vi "cm2nm_write_session_file.vi"(1 "Session Information":T1) -> (0 "NaN/Path/Refnum?":bool)   [LabVIEW 2011]
doc: "Write the session information to xml file, path contained in the field internal field \"CollectionFile\"."
uses:
  cm2nm_sample_set.ctl
  cm2nm_coordinate_information_v2.ctl
  Instrument_type_enum_v2.ctl
  <vilib>/Utility/xml.llb/Write to XML File(string).vi
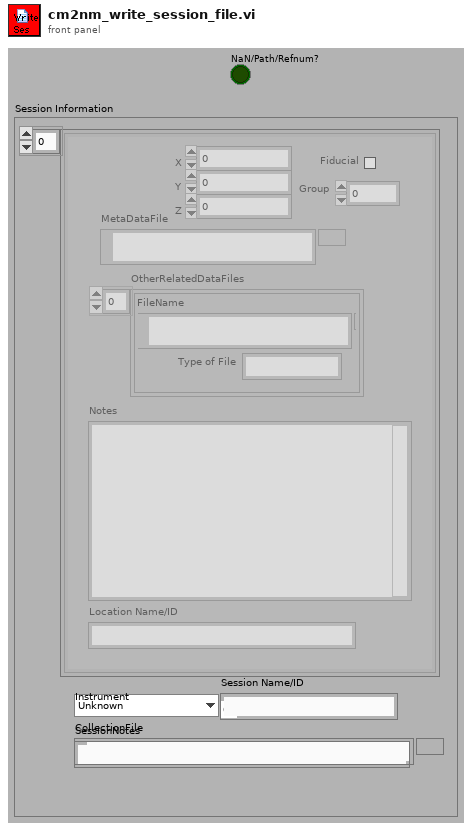
[diagram p1: front panel]
types:
  T1 = typedef "cm2nm_sample_set.ctl" = cluster{"CollectionOfPoints":T2[], "Instrument":T3, "CollectionFile":path, "Session Name/ID":string, "SessionNotes":string}
  T2 = typedef "cm2nm_coordinate_information_v2.ctl" = cluster{"MetaDataFile":path, "X":dbl, "Y":dbl, "Z":dbl, "Group":i32, "Rotation":dbl[unit], "Fiducial":bool, "Magnification":dbl, "Working_Distance":dbl, "Notes":string, "Location Name/ID":string, "OtherRelatedDataFiles":cluster{"Type of File":string, "FileName":path}[], "Available":bool}
  T3 = typedef "Instrument_type_enum_v2.ctl" = enum16{"Unknown", "Philips FEI SEM IRC", "JEOL 7000F EML_MFC", "MXRD MFC", "JEOL_EPMA"}
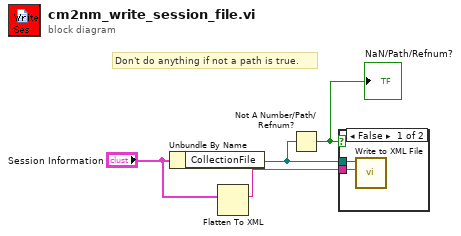
[diagram p0: block diagram]
diagram:
  # "Don't do anything if not a path is true."
  n1 = Unbundle By Name("Session Information") -> ("CollectionFile"=w2:path)
  n2 = Flatten To XML(anything="Session Information") -> (xml string=w3:string)
  n3 = Not A Number/Path/Refnum?(number/path/refnum=w2) -> (NaN/Path/Refnum?=w1:bool)
  "NaN/Path/Refnum?" <- w1
  n4 = case shown="False" w1 {
    tunnel: w3 -> [w6 _]
    tunnel: w2 -> [w5 _]
    frame False {
      n5 = call-poly <vilib>:"Write to XML File.vi"("XML Input"=w6, "XML File Path"=w5) -> ()  [unwired: 3 in, 7 out]
    }
    frame True {
    }
  }
